vi "从数据库获取数据通用可配置(子VI).vi"(8 "错误输入（无错误）":errorcluster, 9 "查询参数数组":string[](array[string])=["CODMn", "CODCr", "DO", "铜", "PH", "氨氮", "比电导率", "水温", "COD", "浊度", "总氮", "总磷", "叶绿素a", "藻密度", "水位", "流速", "瞬时流量", "累积流量", "亚硝酸盐", "硫化物", "ORP", "铅", "镉", "锌", "镍", "锰", "汞"], 10 "table输入":string="实时数据") -> (0 "错误输出":errorcluster, 3 "簇数组":cluster{"待发送数据":string[][]}[][](array[cluster]))   [LabVIEW 2016, in "数据传输系统.lvlib"]
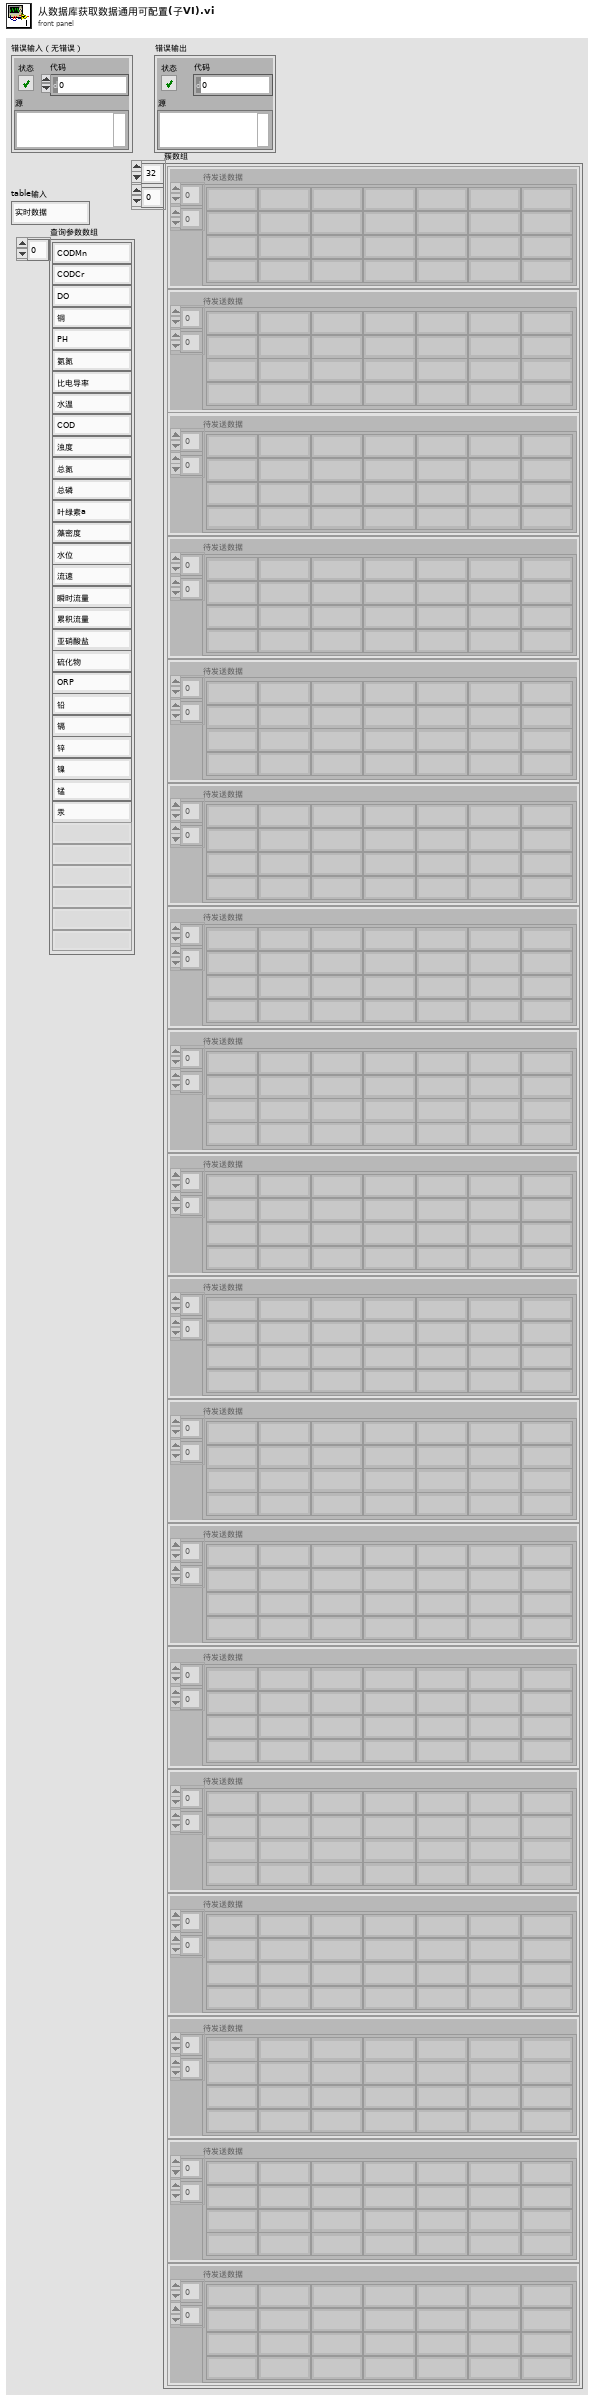
[diagram p1: front panel]
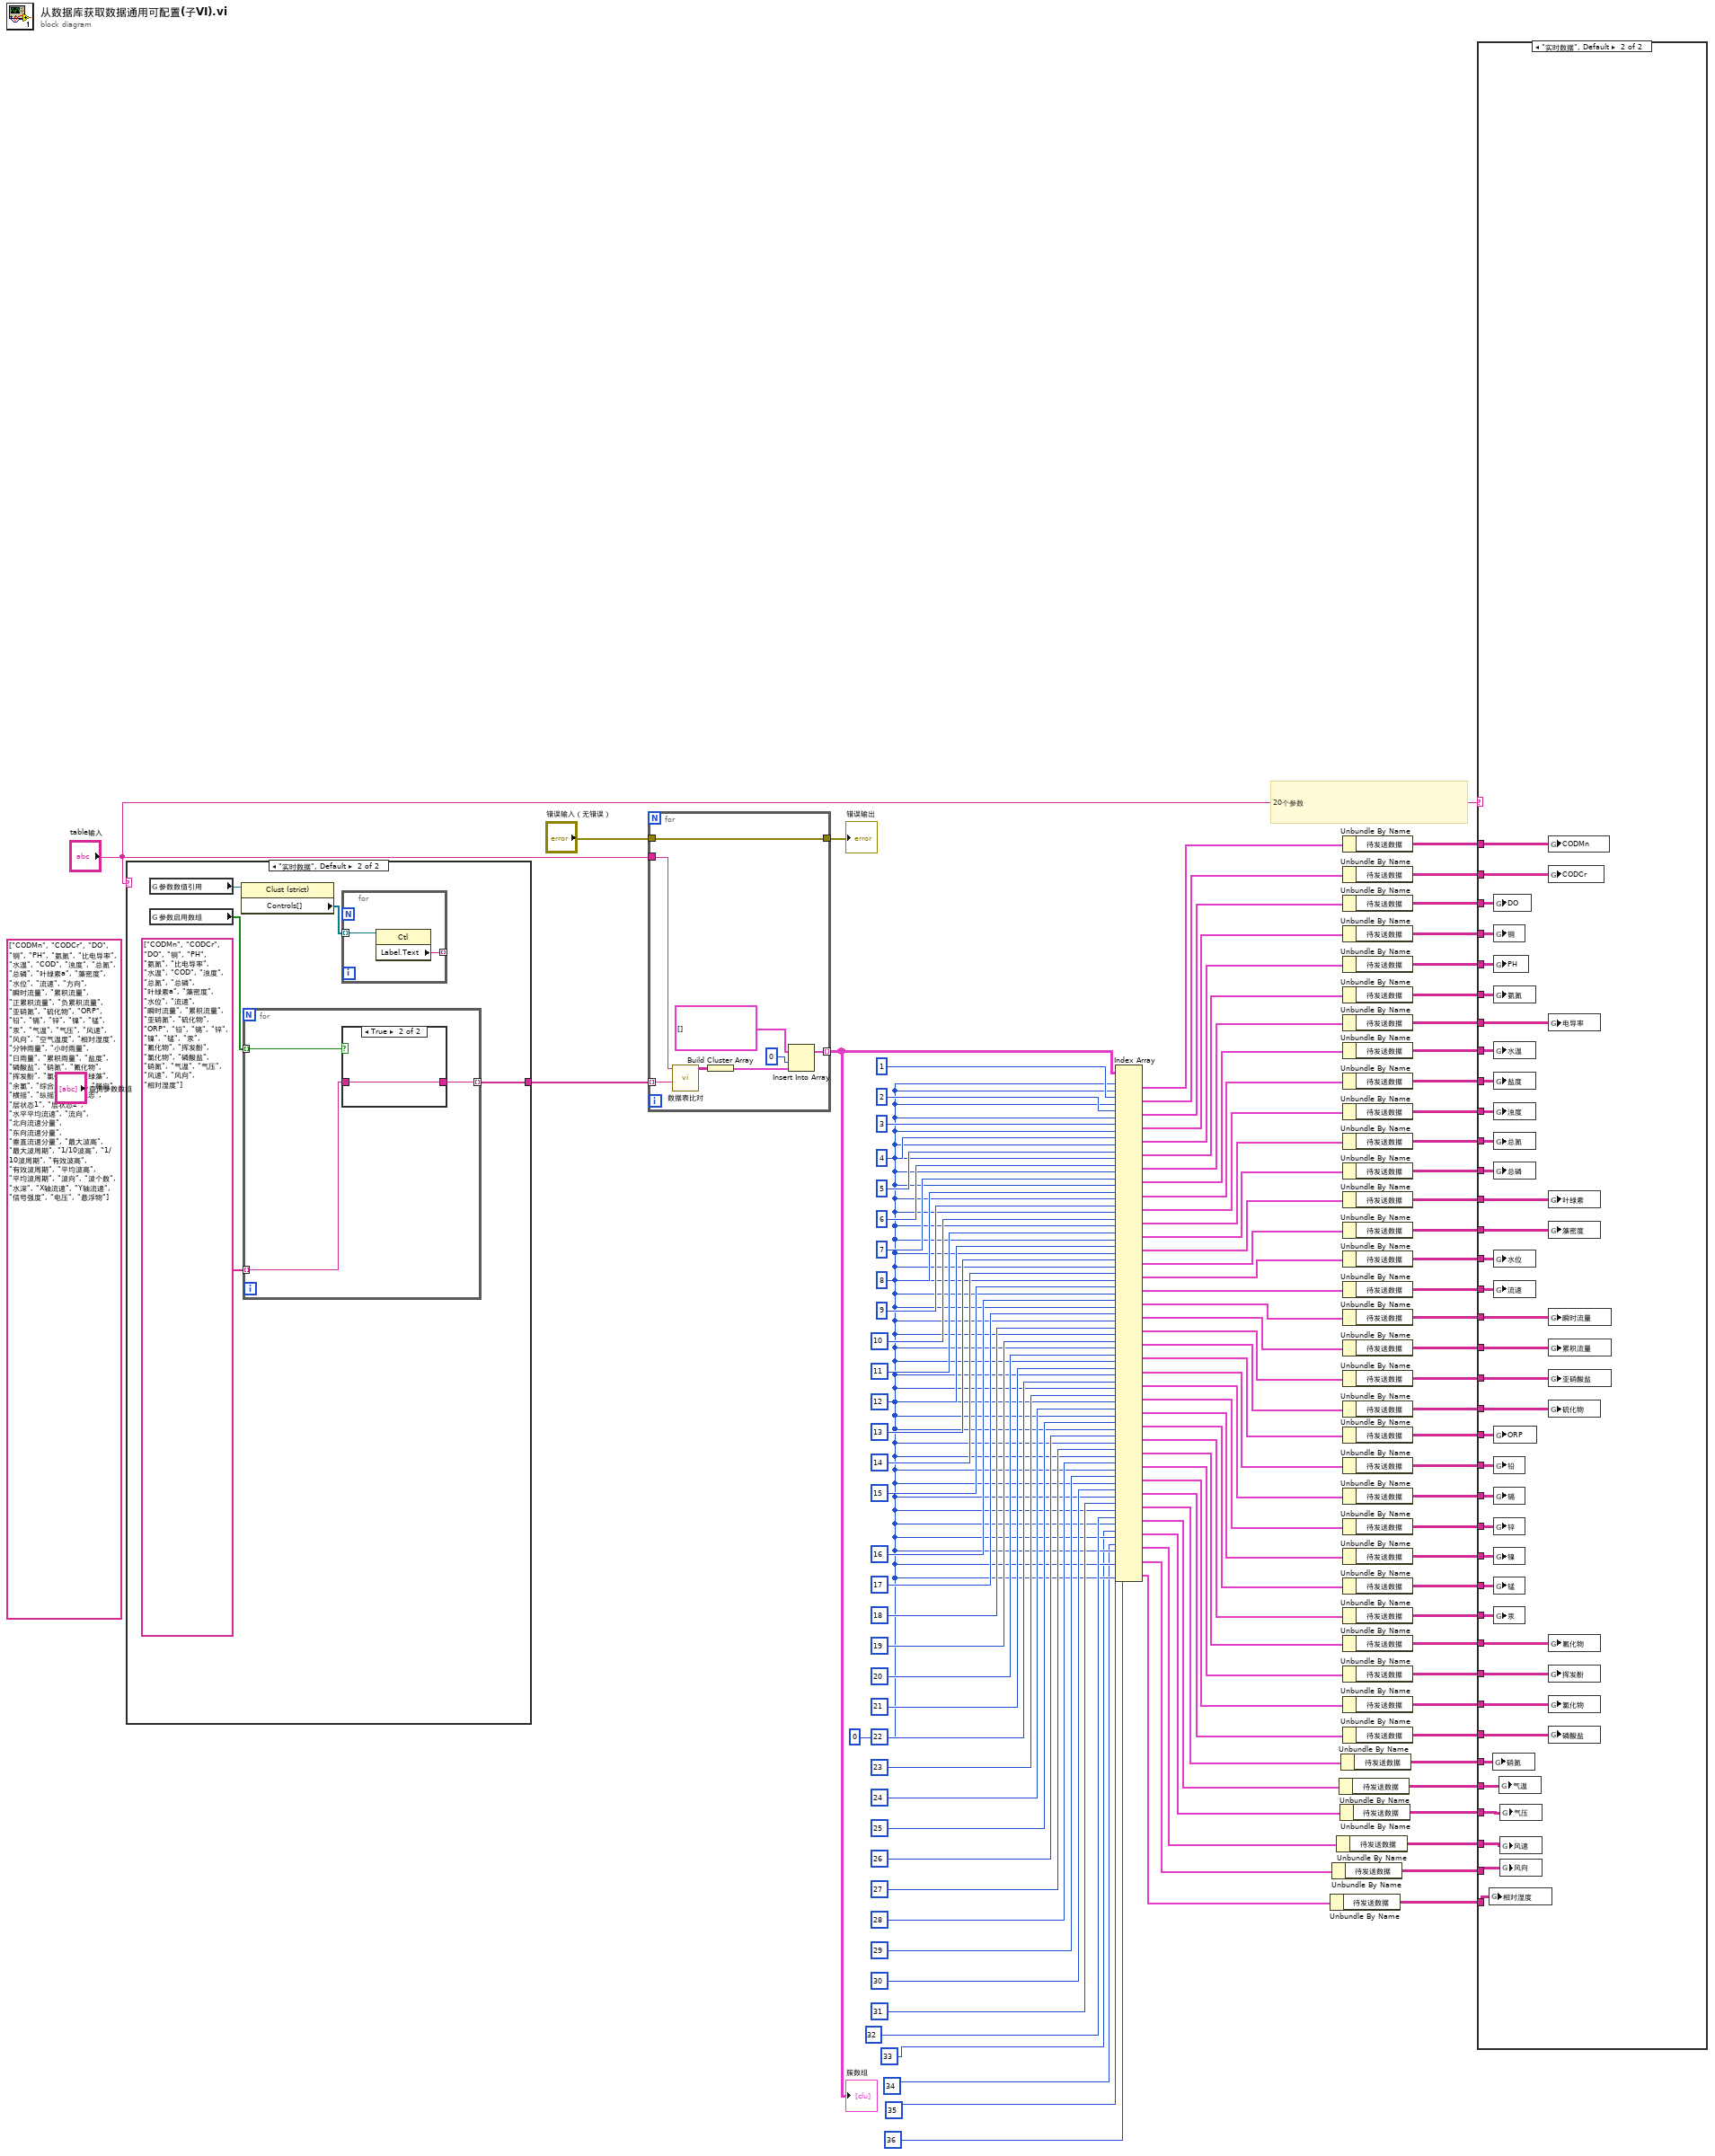
[diagram p0: block diagram]
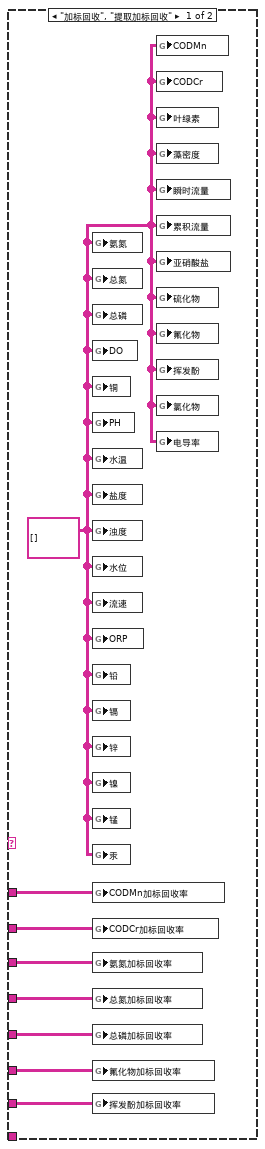
[diagram p2: hidden frame]
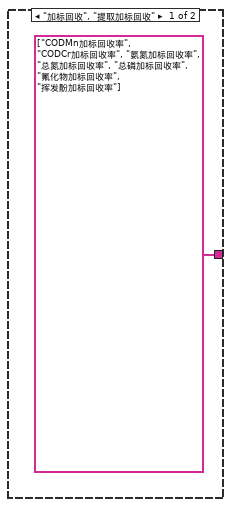
[diagram p3: hidden frame]
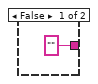
[diagram p4: hidden frame]
diagram:
  (unwired) string[] ["CODMn", "CODCr", "DO", "铜", "PH", "氨氮", "比电导率", "水温", "COD", "浊度", "总氮", "总磷", "叶绿素a", "藻密度", "水位", "流速", "方向", "瞬时流量", "累积流量", "正累积流量", "负累积流量", "亚硝氮", "硫化物", "ORP", "铅", "镉", "锌", "镍", "锰", "汞", "气温", "气压", "风速", "风向", "空气温度", "相对湿度", "分钟雨量", "小时雨量", "日雨量", "累积雨量", "盐度", "磷酸盐", "硝氮", "氟化物", "挥发酚", "氯化物", "蓝绿藻", "余氯", "综合生物毒性", "艏向", "横摇", "纵摇", "分层标志", "层状态1", "层状态2", "水平平均流速", "流向", "北向流速分量", "东向流速分量", "垂直流速分量", "最大波高", "最大波周期", "1/10波高", "1/10波周期", "有效波高", "有效波周期", "平均波高", "平均波周期", "波向", "波个数", "水深", "X轴流速", "Y轴流速", "信号强度", "电压", "悬浮物"] ("Array")
  w5 = 0 ("索引 (行)")
  # "20个参数"
  n1 = case shown="\"实时数据\", Default" "table输入" {
    tunnel: [string[] ["CODMn加标回收率", "CODCr加标回收率", "氨氮加标回收率", "总氮加标回收率", "总磷加标回收率", "氟化物加标回收率", "挥发酚加标回收率"] ("查询参数数组") w121] -> w73
    frame "加标回收", "提取加标回收" {
    }
    frame "实时数据", Default {
      n2 = global read "断电保存全局.vi" "参数数值引用"() -> (w120:refnum<vi>)
      n3 = global read "断电保存全局.vi" "参数启用数组"() -> (w122:bool[])
      n4 = property class="Clust (strict)"(reference=w120) -> ("Controls[]"=w119:refnum<vi>[])  [unwired: 1 in, 2 out]
      n5 = for {
        tunnel: w122 -> [w127] mode=indexing
        tunnel: string[] ["CODMn", "CODCr", "DO", "铜", "PH", "氨氮", "比电导率", "水温", "COD", "浊度", "总氮", "总磷", "叶绿素a", "藻密度", "水位", "流速", "瞬时流量", "累积流量", "亚硝氮", "硫化物", "ORP", "铅", "镉", "锌", "镍", "锰", "汞", "氟化物", "挥发酚", "氯化物", "磷酸盐", "硝氮", "气温", "气压", "风速", "风向", "相对湿度"] ("数组") -> [w126] mode=indexing
        tunnel: [w125] -> w121 mode=indexing
        n6 = case shown="True" w127 {
          tunnel: ["" w129] -> w125
          tunnel: w126 -> [_ w129]
          frame False {
          }
          frame True {
          }
        }
      }
      n7 = for {
        tunnel: w119 -> [w124] mode=indexing
        tunnel: [w123] -> _ mode=indexing
        n8 = property class="Ctl"(reference=w124) -> ("Label.Text"=w123:string)  [unwired: 1 in, 2 out]
      }
    }
  }
  n9 = for {
    tunnel: w73 -> [w131] mode=indexing
    tunnel: [w135] -> w115 mode=indexing
    tunnel: "table输入" -> [w132]
    tunnel: [w130] -> w116
    tunnel: "错误输入（无错误）" -> [w130]
    n10 = call "数据表比对.vi"("查询元素输入"=w131, "table输入"=w132) -> ("待发送数据"=w137:string[][])  [unwired: 6 in, 3 out]
    n11 = Build Cluster Array(w137) -> (w136:cluster{"待发送数据":string[][]}[])
    n12 = Insert Into Array(array=cluster{"待发送数据":string[][]}[] [] ("簇数组"), index=0 ("索引"), new element=w136) -> (w135:cluster{"待发送数据":string[][]}[])
  }
  "簇数组" <- w115
  "错误输出" <- w116
  n13 = Index Array(array=w115, index (row) #1=w5, index (col) #1=w5, index (row) #2=1 ("索引 (行)"), index (col) #2=w5, index (row) #3=2 ("索引 (行)"), index (col) #3=w5, index (row) #4=3 ("索引 (行)"), index (col) #4=w5, index (row) #5=4 ("索引 (行)"), index (col) #5=w5, index (row) #6=5 ("索引 (行)"), index (col) #6=w5, index (row) #7=6 ("索引 (行)"), index (col) #7=w5, index (row) #8=7 ("索引 (行)"), index (col) #8=w5, index (row) #9=8 ("索引 (行)"), index (col) #9=w5, index (row) #10=9 ("索引 (行)"), index (col) #10=w5, index (row) #11=10 ("索引 (行)"), index (col) #11=w5, index (row) #12=11 ("索引 (行)"), index (col) #12=w5, index (row) #13=12 ("索引 (行)"), index (col) #13=w5, index (row) #14=13 ("索引 (行)"), index (col) #14=w5, index (row) #15=14 ("禁用的索引 (行)"), index (col) #15=w5, index (row) #16=15 ("禁用的索引 (行)"), index (col) #16=w5, index (row) #17=16 ("禁用的索引 (行)"), index (col) #17=w5, index (row) #18=17 ("禁用的索引 (行)"), index (col) #18=w5, index (row) #19=18 ("禁用的索引 (行)"), index (col) #19=w5, index (row) #20=19 ("禁用的索引 (行)"), index (col) #20=w5, index (row) #21=20 ("禁用的索引 (行)"), index (col) #21=w5, index (row) #22=21 ("禁用的索引 (行)"), index (col) #22=w5, index (row) #23=22 ("禁用的索引 (行)"), index (col) #23=w5, index (row) #24=23 ("禁用的索引 (行)"), index (col) #24=w5, index (row) #25=24 ("禁用的索引 (行)"), index (col) #25=w5, index (row) #26=25 ("禁用的索引 (行)"), index (col) #26=w5, index (row) #27=26 ("禁用的索引 (行)"), index (col) #27=w5, index (row) #28=27 ("禁用的索引 (行)"), index (col) #28=w5, index (row) #29=28 ("禁用的索引 (行)"), index (col) #29=w5, index (row) #30=29 ("禁用的索引 (行)"), index (col) #30=w5, index (row) #31=30 ("索引 (行)"), index (col) #31=w5, index (row) #32=31 ("索引 (行)"), index (col) #32=w5, index (row) #33=32 ("disabled index (row)"), index (col) #33=w5, index (row) #34=33 ("disabled index (row)"), index (col) #34=w5, index (row) #35=34 ("disabled index (row)"), index (col) #35=w5, index (row) #36=35 ("disabled index (row)"), index (col) #36=w5, index (row) #37=36 ("disabled index (row)"), index (col) #37=w5) -> (element #1=w114:cluster{"待发送数据":string[][]}, element #2=w99:cluster{"待发送数据":string[][]}, element #3=w98:cluster{"待发送数据":string[][]}, element #4=w97:cluster{"待发送数据":string[][]}, element #5=w96:cluster{"待发送数据":string[][]}, element #6=w95:cluster{"待发送数据":string[][]}, element #7=w93:cluster{"待发送数据":string[][]}, element #8=w94:cluster{"待发送数据":string[][]}, element #9=w92:cluster{"待发送数据":string[][]}, element #10=w91:cluster{"待发送数据":string[][]}, element #11=w90:cluster{"待发送数据":string[][]}, element #12=w89:cluster{"待发送数据":string[][]}, element #13=w88:cluster{"待发送数据":string[][]}, element #14=w87:cluster{"待发送数据":string[][]}, element #15=w68:cluster{"待发送数据":string[][]}, element #16=w66:cluster{"待发送数据":string[][]}, element #17=w65:cluster{"待发送数据":string[][]}, element #18=w64:cluster{"待发送数据":string[][]}, element #19=w59:cluster{"待发送数据":string[][]}, element #20=w55:cluster{"待发送数据":string[][]}, element #21=w54:cluster{"待发送数据":string[][]}, element #22=w47:cluster{"待发送数据":string[][]}, element #23=w46:cluster{"待发送数据":string[][]}, element #24=w45:cluster{"待发送数据":string[][]}, element #25=w39:cluster{"待发送数据":string[][]}, element #26=w37:cluster{"待发送数据":string[][]}, element #27=w36:cluster{"待发送数据":string[][]}, element #28=w31:cluster{"待发送数据":string[][]}, element #29=w26:cluster{"待发送数据":string[][]}, element #30=w25:cluster{"待发送数据":string[][]}, element #31=w20:cluster{"待发送数据":string[][]}, element #32=w17:cluster{"待发送数据":string[][]}, element #33=w16:cluster{"待发送数据":string[][]}, element #34=w15:cluster{"待发送数据":string[][]}, element #35=w14:cluster{"待发送数据":string[][]}, element #36=w13:cluster{"待发送数据":string[][]}, element #37=w12:cluster{"待发送数据":string[][]})
  n14 = Unbundle By Name(w12) -> ("待发送数据"=w7:string[][])
  n15 = Unbundle By Name(w13) -> ("待发送数据"=w8:string[][])
  n16 = Unbundle By Name(w14) -> ("待发送数据"=w9:string[][])
  n17 = Unbundle By Name(w16) -> ("待发送数据"=w11:string[][])
  n18 = Unbundle By Name(w15) -> ("待发送数据"=w10:string[][])
  n19 = Unbundle By Name(w17) -> ("待发送数据"=w18:string[][])
  n20 = Unbundle By Name(w114) -> ("待发送数据"=w113:string[][])
  n21 = Unbundle By Name(w99) -> ("待发送数据"=w86:string[][])
  n22 = Unbundle By Name(w98) -> ("待发送数据"=w85:string[][])
  n23 = Unbundle By Name(w97) -> ("待发送数据"=w84:string[][])
  n24 = Unbundle By Name(w96) -> ("待发送数据"=w83:string[][])
  n25 = Unbundle By Name(w95) -> ("待发送数据"=w82:string[][])
  n26 = Unbundle By Name(w93) -> ("待发送数据"=w81:string[][])
  n27 = Unbundle By Name(w94) -> ("待发送数据"=w80:string[][])
  n28 = Unbundle By Name(w92) -> ("待发送数据"=w79:string[][])
  n29 = Unbundle By Name(w91) -> ("待发送数据"=w78:string[][])
  n30 = Unbundle By Name(w90) -> ("待发送数据"=w77:string[][])
  n31 = Unbundle By Name(w89) -> ("待发送数据"=w76:string[][])
  n32 = Unbundle By Name(w88) -> ("待发送数据"=w74:string[][])
  n33 = Unbundle By Name(w87) -> ("待发送数据"=w75:string[][])
  n34 = Unbundle By Name(w68) -> ("待发送数据"=w67:string[][])
  n35 = Unbundle By Name(w66) -> ("待发送数据"=w63:string[][])
  n36 = Unbundle By Name(w65) -> ("待发送数据"=w62:string[][])
  n37 = Unbundle By Name(w64) -> ("待发送数据"=w61:string[][])
  n38 = Unbundle By Name(w59) -> ("待发送数据"=w53:string[][])
  n39 = Unbundle By Name(w55) -> ("待发送数据"=w52:string[][])
  n40 = Unbundle By Name(w54) -> ("待发送数据"=w51:string[][])
  n41 = Unbundle By Name(w47) -> ("待发送数据"=w44:string[][])
  n42 = Unbundle By Name(w46) -> ("待发送数据"=w43:string[][])
  n43 = Unbundle By Name(w45) -> ("待发送数据"=w42:string[][])
  n44 = Unbundle By Name(w39) -> ("待发送数据"=w38:string[][])
  n45 = Unbundle By Name(w37) -> ("待发送数据"=w35:string[][])
  n46 = Unbundle By Name(w36) -> ("待发送数据"=w34:string[][])
  n47 = Unbundle By Name(w31) -> ("待发送数据"=w30:string[][])
  n48 = Unbundle By Name(w26) -> ("待发送数据"=w24:string[][])
  n49 = Unbundle By Name(w25) -> ("待发送数据"=w23:string[][])
  n50 = Unbundle By Name(w20) -> ("待发送数据"=w19:string[][])
  n51 = case shown="\"实时数据\", Default" "table输入" {
    tunnel: w113 -> [w145 w182]
    tunnel: w86 -> [w144 w181]
    tunnel: w85 -> [w143 w180]
    tunnel: w84 -> [w142 w179]
    tunnel: w83 -> [w141 w178]
    tunnel: w82 -> [w140 w177]
    tunnel: w81 -> [w139 w176]
    tunnel: w80 -> [_ w175]
    tunnel: w79 -> [_ w174]
    tunnel: w78 -> [_ w173]
    tunnel: w77 -> [_ w172]
    tunnel: w76 -> [_ w171]
    tunnel: w75 -> [_ w170]
    tunnel: w74 -> [_ w169]
    tunnel: w67 -> [_ w168]
    tunnel: w63 -> [_ w167]
    tunnel: w62 -> [_ w166]
    tunnel: w61 -> [_ w165]
    tunnel: w53 -> [_ w164]
    tunnel: w52 -> [_ w163]
    tunnel: w51 -> [_ w162]
    tunnel: w44 -> [_ w161]
    tunnel: w43 -> [_ w160]
    tunnel: w42 -> [_ w159]
    tunnel: w38 -> [_ w158]
    tunnel: w35 -> [_ w157]
    tunnel: w34 -> [_ w156]
    tunnel: w30 -> [_ w155]
    tunnel: w24 -> [_ w154]
    tunnel: w23 -> [_ w153]
    tunnel: w19 -> [_ w152]
    tunnel: w18 -> [_ w151]
    tunnel: w11 -> [_ w150]
    tunnel: w10 -> [_ w149]
    tunnel: w9 -> [_ w146]
    tunnel: w8 -> [_ w148]
    tunnel: w7 -> [_ w147]
    frame "加标回收", "提取加标回收" {
      w138 = string[][] [] ("DO")
      n52 = global write "全局 所有参数.vi" "氨氮"(w138) -> ()
      n53 = global write "全局 所有参数.vi" "总氮"(w138) -> ()
      n54 = global write "全局 所有参数.vi" "总磷"(w138) -> ()
      n55 = global write "全局 所有参数.vi" "DO"(w138) -> ()
      n56 = global write "全局 所有参数.vi" "铜"(w138) -> ()
      n57 = global write "全局 所有参数.vi" "PH"(w138) -> ()
      n58 = global write "全局 所有参数.vi" "水温"(w138) -> ()
      n59 = global write "全局 所有参数.vi" "盐度"(w138) -> ()
      n60 = global write "全局 所有参数.vi" "浊度"(w138) -> ()
      n61 = global write "全局 所有参数.vi" "水位"(w138) -> ()
      n62 = global write "全局 所有参数.vi" "流速"(w138) -> ()
      n63 = global write "全局 所有参数.vi" "ORP"(w138) -> ()
      n64 = global write "全局 所有参数.vi" "铅"(w138) -> ()
      n65 = global write "全局 所有参数.vi" "镉"(w138) -> ()
      n66 = global write "全局 所有参数.vi" "锌"(w138) -> ()
      n67 = global write "全局 所有参数.vi" "镍"(w138) -> ()
      n68 = global write "全局 所有参数.vi" "锰"(w138) -> ()
      n69 = global write "全局 所有参数.vi" "汞"(w138) -> ()
      n70 = global write "全局 所有参数.vi" "CODMn加标回收率"(w145) -> ()
      n71 = global write "全局 所有参数.vi" "CODCr加标回收率"(w144) -> ()
      n72 = global write "全局 所有参数.vi" "氨氮加标回收率"(w143) -> ()
      n73 = global write "全局 所有参数.vi" "总氮加标回收率"(w142) -> ()
      n74 = global write "全局 所有参数.vi" "总磷加标回收率"(w141) -> ()
      n75 = global write "全局 所有参数.vi" "氟化物加标回收率"(w140) -> ()
      n76 = global write "全局 所有参数.vi" "挥发酚加标回收率"(w139) -> ()
      n77 = global write "全局 所有参数.vi" "CODMn"(w138) -> ()
      n78 = global write "全局 所有参数.vi" "CODCr"(w138) -> ()
      n79 = global write "全局 所有参数.vi" "叶绿素"(w138) -> ()
      n80 = global write "全局 所有参数.vi" "藻密度"(w138) -> ()
      n81 = global write "全局 所有参数.vi" "瞬时流量"(w138) -> ()
      n82 = global write "全局 所有参数.vi" "累积流量"(w138) -> ()
      n83 = global write "全局 所有参数.vi" "亚硝酸盐"(w138) -> ()
      n84 = global write "全局 所有参数.vi" "硫化物"(w138) -> ()
      n85 = global write "全局 所有参数.vi" "氟化物"(w138) -> ()
      n86 = global write "全局 所有参数.vi" "挥发酚"(w138) -> ()
      n87 = global write "全局 所有参数.vi" "氯化物"(w138) -> ()
      n88 = global write "全局 所有参数.vi" "电导率"(w138) -> ()
    }
    frame "实时数据", Default {
      n89 = global write "全局 所有参数.vi" "相对湿度"(w147) -> ()
      n90 = global write "全局 所有参数.vi" "硝氮"(w151) -> ()
      n91 = global write "全局 所有参数.vi" "DO"(w180) -> ()
      n92 = global write "全局 所有参数.vi" "铜"(w179) -> ()
      n93 = global write "全局 所有参数.vi" "PH"(w178) -> ()
      n94 = global write "全局 所有参数.vi" "氨氮"(w177) -> ()
      n95 = global write "全局 所有参数.vi" "水温"(w175) -> ()
      n96 = global write "全局 所有参数.vi" "盐度"(w174) -> ()
      n97 = global write "全局 所有参数.vi" "浊度"(w173) -> ()
      n98 = global write "全局 所有参数.vi" "总氮"(w172) -> ()
      n99 = global write "全局 所有参数.vi" "总磷"(w171) -> ()
      n100 = global write "全局 所有参数.vi" "水位"(w168) -> ()
      n101 = global write "全局 所有参数.vi" "流速"(w167) -> ()
      n102 = global write "全局 所有参数.vi" "ORP"(w162) -> ()
      n103 = global write "全局 所有参数.vi" "铅"(w161) -> ()
      n104 = global write "全局 所有参数.vi" "镉"(w160) -> ()
      n105 = global write "全局 所有参数.vi" "锌"(w159) -> ()
      n106 = global write "全局 所有参数.vi" "镍"(w158) -> ()
      n107 = global write "全局 所有参数.vi" "锰"(w157) -> ()
      n108 = global write "全局 所有参数.vi" "汞"(w156) -> ()
      n109 = global write "全局 所有参数.vi" "气温"(w150) -> ()
      n110 = global write "全局 所有参数.vi" "气压"(w149) -> ()
      n111 = global write "全局 所有参数.vi" "风速"(w146) -> ()
      n112 = global write "全局 所有参数.vi" "风向"(w148) -> ()
      n113 = global write "全局 所有参数.vi" "CODMn"(w182) -> ()
      n114 = global write "全局 所有参数.vi" "CODCr"(w181) -> ()
      n115 = global write "全局 所有参数.vi" "电导率"(w176) -> ()
      n116 = global write "全局 所有参数.vi" "叶绿素"(w169) -> ()
      n117 = global write "全局 所有参数.vi" "藻密度"(w170) -> ()
      n118 = global write "全局 所有参数.vi" "瞬时流量"(w166) -> ()
      n119 = global write "全局 所有参数.vi" "累积流量"(w165) -> ()
      n120 = global write "全局 所有参数.vi" "亚硝酸盐"(w164) -> ()
      n121 = global write "全局 所有参数.vi" "硫化物"(w163) -> ()
      n122 = global write "全局 所有参数.vi" "氟化物"(w155) -> ()
      n123 = global write "全局 所有参数.vi" "挥发酚"(w154) -> ()
      n124 = global write "全局 所有参数.vi" "氯化物"(w153) -> ()
      n125 = global write "全局 所有参数.vi" "磷酸盐"(w152) -> ()
    }
  }
